vi "GA_Mutate.vi"(6 "Parameters":T1={"Population size"=100, "Generations no."=500, "Crossover probabality"=6.0, "Mutation mode"=enum."one-point, fitness-adjustable rate", "Creep mutation"=FALSE, "Mutation rate"=0.005, "Min mutation rate"=0.005, "Max mutation rate"=0.0005, "Relative fitness differential"=0.25, "Reproduction plan"=enum."Steady-state-replace-random", "Elitism"=FALSE, "FeaturesPerChannel"=0} {"Relative fitness differential" min=0.0 max=1.0; "Max mutation rate" min=0.0 max=1.0; "Min mutation rate" min=0.0 max=1.0; "Mutation rate" min=0.0 max=1.0; "Crossover probabality" min=0.0 max=1.0; "Generations no." min=1; "Population size" min=1}, 11 "Genotype in":i8[](array[numeric])) -> (3 "Genotype out":i8[](array[numeric]))   [LabVIEW 2016, in "GA.lvlib"]
doc: "Mutates genotype in way defined by parameters"
uses:
  GA.lvlib
  GA_tParameters.ctl
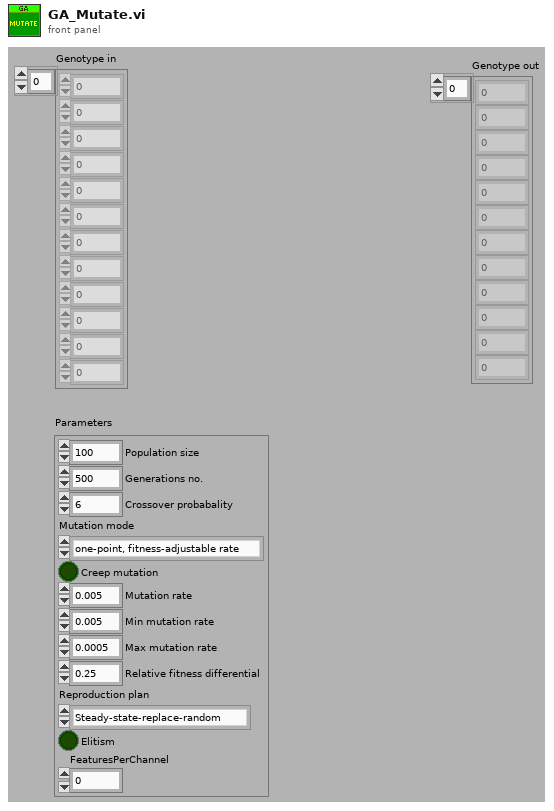
[diagram p1: front panel]
types:
  T1 = typedef "GA.lvlib/GA_tParameters.ctl" = cluster{"Population size":i32, "Generations no.":i32, "Crossover probabality":dbl, "Mutation mode":enum16{"one-point, fixed rate", "one-point, fitness-adjustable rate", "one-point, distance-adjustable rate"}, "Creep mutation":bool, "Mutation rate":dbl, "Min mutation rate":dbl, "Max mutation rate":dbl, "Relative fitness differential":dbl, "Reproduction plan":enum16{"Full generational replacement", "Steady-state-replace-random", "Steady-state-replace-worst"}, "Elitism":bool, "FeaturesPerChannel":i32}
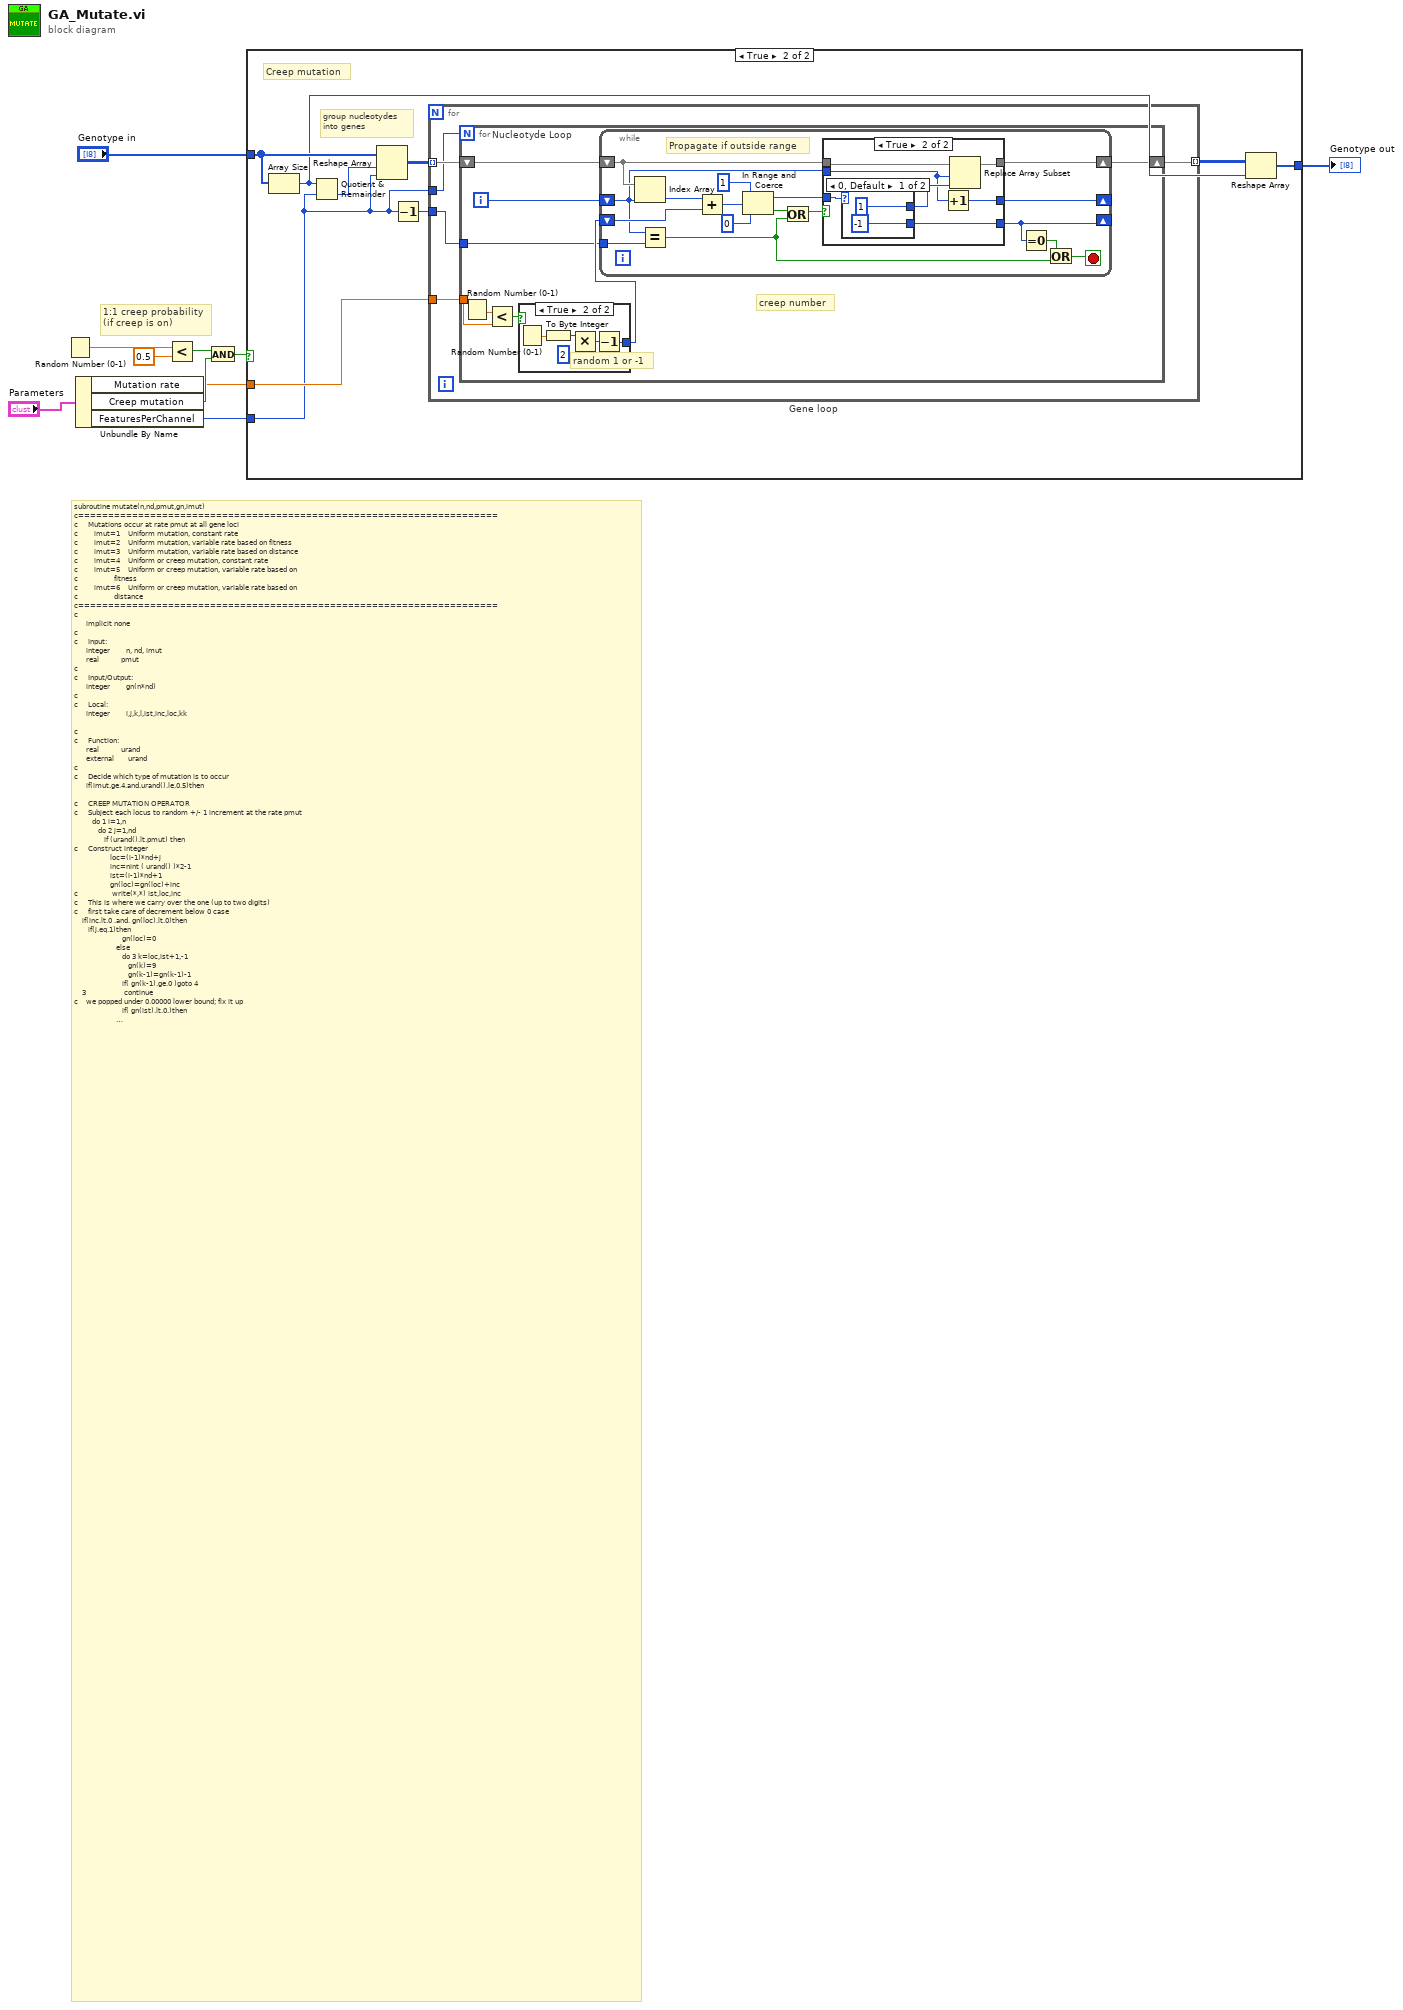
[diagram p0: block diagram]
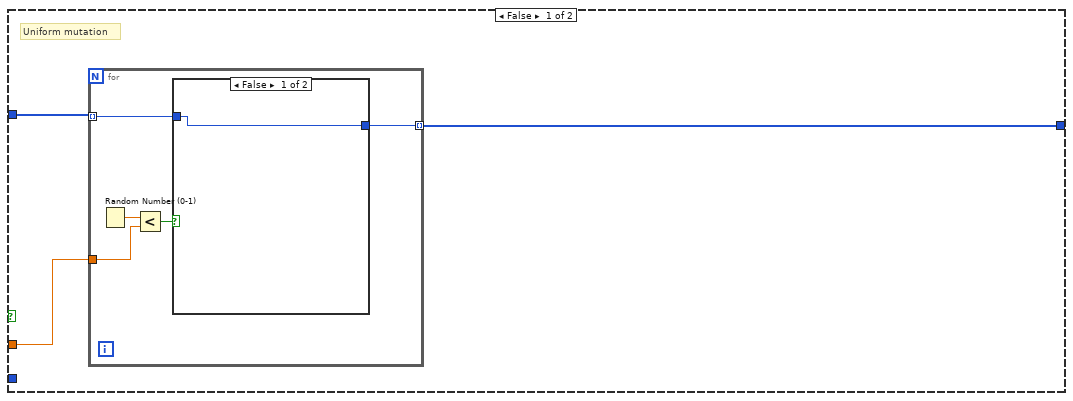
[diagram p2: hidden frame]
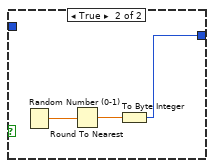
[diagram p3: hidden frame]
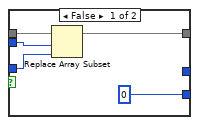
[diagram p4: hidden frame]
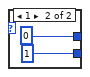
[diagram p5: hidden frame]
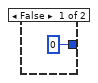
[diagram p6: hidden frame]
diagram:
  # "1:1 creep probability\n(if creep is on)"
  # "subroutine mutate(n,nd,pmut,gn,imut)\nc======================================================================\nc     Mutations occur at rate pmut at all gene loci\nc        imut=1    Uniform mutation, constant rate\nc        imut=2    Uniform mutation, variable rate based on fitness\nc        imut=3    Uniform mutation, variable rate based on distance\nc        imut=4    Uniform or creep mutation, constant rate\nc        imut=5    Uniform or creep mutation, variable rate based on\nc                  fitness\nc        imut=6    Uniform or creep mutation, variable rate based on\nc                  distance\nc======================================================================\nc\n      implicit none\nc\nc     Input:\n      integer        n, nd, imut\n      real           pmut\nc\nc     Input/Output:\n      integer        gn(n*nd)\nc\nc     Local:\n      integer        i,j,k,l,ist,inc,loc,kk\n\nc\nc     Function:\n      real           urand\n      external       urand\nc\nc     Decide which type of mutation is to occur\n      if(imut.ge.4.and.urand().le.0.5)then\n\nc     CREEP MUTATION OPERATOR\nc     Subject each locus to random +/- 1 increment at the rate pmut\n         do 1 i=1,n\n            do 2 j=1,nd\n               if (urand().lt.pmut) then\nc     Construct integer\n                  loc=(i-1)*nd+j\n                  inc=nint ( urand() )*2-1\n                  ist=(i-1)*nd+1\n                  gn(loc)=gn(loc)+inc\nc                 write(*,*) ist,loc,inc\nc     This is where we carry over the one (up to two digits)\nc     first take care of decrement below 0 case\n\t\t  if(inc.lt.0 .and. gn(loc).lt.0)then\n\t\t     if(j.eq.1)then\n                        gn(loc)=0\n                     else\n                        do 3 k=loc,ist+1,-1\n                           gn(k)=9\n                           gn(k-1)=gn(k-1)-1\n                        if( gn(k-1).ge.0 )goto 4\n    3                   continue\nc    we popped under 0.00000 lower bound; fix it up\n                        if( gn(ist).lt.0.)then\n                           do 5 l=ist,loc\n                              gn(l)=0\n    5                      continue\n                        endif\n    4                   continue\n                     endif\n                  endif\n                  if(inc.gt.0 .and. gn(loc).gt.9)then\n                     if(j.eq.1)then\n                        gn(loc)=9\n                     else\n                        do 6 k=loc,ist+1,-1\n                           gn(k)=0\n                           gn(k-1)=gn(k-1)+1\n                           if( gn(k-1).le.9 )goto 7\n    6                   continue\nc                       we popped over 9.99999 upper bound; fix it up\n                       if( gn(ist).gt.9 )then\n                           do 8 l=ist,loc\n                              gn(l)=9\n    8                      continue\n                        endif\n    7                   continue\n                     endif\n                  endif\n               endif\n    2       continue\n    1    continue\n\n      else\n\nc     UNIFORM MUTATION OPERATOR\nc     Subject each locus to random mutation at the rate pmut\n         do 10 i=1,n*nd\n            if (urand().lt.pmut) then\n               gn(i)=int(urand()*10.)\n            endif\n   10    continue\n      endif\n\n      return\n      end"
  n1 = Random Number (0-1)() -> (number: 0 to 1=w10:dbl)
  n2 = Unbundle By Name("Parameters") -> ("Mutation rate"=w2:dbl, "Creep mutation"=w6:bool, "FeaturesPerChannel"=w3:i32)
  n3 = Less?(x=w10, y=0.5) -> (x < y?=w7:bool)
  n4 = And(x=w7, y=w6) -> (x .and. y?=w5:bool)
  n5 = case shown="True" w5 {
    tunnel: "Genotype in" -> [w13 w31]
    tunnel: w3 -> [_ w24]
    tunnel: w2 -> [w12 w28]
    tunnel: [w11 w23] -> w1
    frame False {
      # "Uniform mutation"
      n6 = for {
        tunnel: w13 -> [w15] mode=indexing
        tunnel: w12 -> [w17]
        tunnel: [w14] -> w11 mode=indexing
        n7 = Random Number (0-1)() -> (number: 0 to 1=w18:dbl)
        n8 = Less?(x=w18, y=w17) -> (x < y?=w16:bool)
        n9 = case shown="False" w16 {
          tunnel: w15 -> [w19 _]
          tunnel: [w19 w20] -> w14
          frame False {
          }
          frame True {
            n10 = Random Number (0-1)() -> (number: 0 to 1=w21:dbl)
            n11 = Round To Nearest(number=w21) -> (nearest integer value=w22:dbl)
            n12 = To Byte Integer(number=w22) -> (8bit integer=w20:i8)
          }
        }
      }
    }
    frame True {
      # "group nucleotydes\ninto genes"
      # "Creep mutation"
      n13 = Array Size(array=w31) -> (size(s)=w26:i32)
      n14 = Quotient & Remainder(x=w26, y=w24) -> (floor(x/y)=w30:i32)  [unwired: 1 out]
      n15 = Reshape Array(w31, w30, w24) -> (w29:i8[][])
      n16 = Decrement(x=w24) -> (x-1=w25:i32)
      n17 = for "Gene loop" {
        tunnel: w29 -> [w36] mode=indexing
        tunnel: w25 -> [w34]
        tunnel: w28 -> [w35]
        tunnel: [w33] -> w27 mode=indexing
        tunnel: w24 -> [w32]
        n18 = for "Nucleotyde Loop" {
          N: w32 -> [_]
          shift-right: [w37] -> w33
          shift-left: w36 -> [w41]
          tunnel: w35 -> [w42]
          tunnel: w34 -> [w38]
          i -> [w39]
          # "random 1 or -1"
          # "creep number"
          n19 = Random Number (0-1)() -> (number: 0 to 1=w44:dbl)
          n20 = Less?(x=w44, y=w42) -> (x < y?=w43:bool)
          n21 = case shown="True" w43 {
            tunnel: [i8 0 ("y") w79] -> w40
            frame False {
            }
            frame True {
              n22 = Random Number (0-1)() -> (number: 0 to 1=w82:dbl)
              n23 = To Byte Integer(number=w82) -> (8bit integer=w81:i8)
              n24 = Multiply(x=w81, y=i8 2) -> (x*y=w80:i8)
              n25 = Decrement(x=w80) -> (x-1=w79:i8)
            }
          }
          n26 = while {
            shift-right: [w51] -> _
            shift-left: w39 -> [w46]
            shift-right: [w52] -> _
            shift-left: w40 -> [w60]
            tunnel: w38 -> [w61]
            shift-right: [w53] -> w37
            shift-left: w41 -> [w55]
            stop <- w56 stop-if-true
            # "Propagate if outside range"
            n27 = Index Array(array=w55, index=w46) -> (element=w45:i8)
            n28 = Equal?(x=w46, y=w61) -> (x = y?=w49:bool)
            n29 = Add(x=w45, y=w60) -> (x+y=w59:i8)
            n30 = In Range and Coerce(upper limit=i8 1 ("lower limit"), x=w59, lower limit=i8 0) -> (coerced(x)=w54:i8, In Range?=w47:bool)
            n31 = Or(x=w47, y=w49) -> (x .or. y?=w48:bool)
            n32 = case shown="True" w48 {
              tunnel: w55 -> [w66 w72]
              tunnel: w46 -> [w65 w68]
              tunnel: w54 -> [w64 w73]
              tunnel: [w63 w71] -> w53
              tunnel: [i8 0 ("lower limit") w70] -> w52
              tunnel: [_ w67] -> w51
              frame False {
                n33 = Replace Array Subset(array=w66, new element=w64, index=w65) -> (w63:i8[])
              }
              frame True {
                n34 = case shown="0, Default" w73 {
                  tunnel: [i8 1 ("lower limit") i8 0 ("lower limit")] -> w69
                  tunnel: [i8 -1 ("lower limit") i8 1 ("lower limit")] -> w70
                  frame 0, Default {
                  }
                  frame 1 {
                  }
                }
                n35 = Increment(x=w68) -> (x+1=w67:i32)
                n36 = Replace Array Subset(array=w72, new element=w69, index=w68) -> (w71:i8[])
              }
            }
            n37 = Equal To 0?(x=w52) -> (x = 0?=w50:bool)
            n38 = Or(x=w50, y=w49) -> (x .or. y?=w56:bool)
          }
        }
      }
      n39 = Reshape Array(w27, w26) -> (w23:i8[])
    }
  }
  "Genotype out" <- w1
